vi "StiffnessTest.vi"(8 "error in (no error)":errorcluster, 10 "Model in":refnum<class "Model.lvclass">, 11 "Test Actuator State in":refnum<class "Test Actuator State.lvclass">) -> (0 "error out":errorcluster, 2 "Model out":refnum<class "Model.lvclass">, 3 "Test Actuator State out":refnum<class "Test Actuator State.lvclass">)   [LabVIEW 2016, in "Test Actuator State.lvclass"]
uses:
  Test Actuator State.lvclass
  Model/Model/Model.lvclass
  Typedefs/TestStatus.ctl
  Model/Model/Model.lvclass/Model.ctl
  Typedefs/HPMT_Typedefs.lvlib
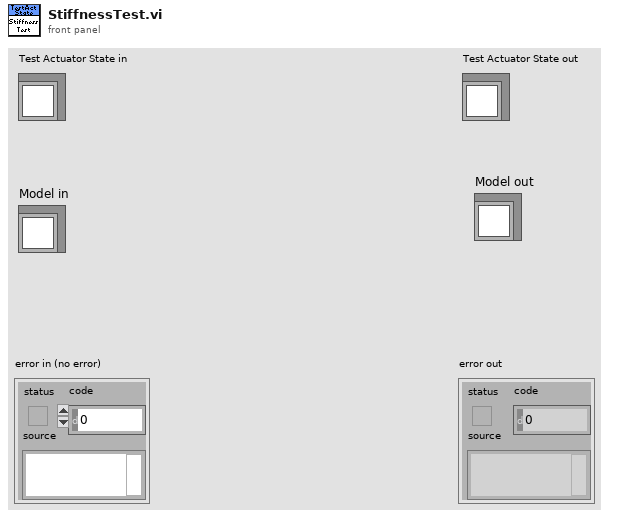
[diagram p1: front panel]
types:
  T1 = typedef "HPMT_Typedefs.lvlib/TestStatus.ctl" = enum16{"Not Run", "Running", "Passed", "Failed"}
  T2 = typedef "HPMT_Typedefs.lvlib/AllTestStatus.ctl" = cluster{"Stiffness Test":T1}
  T3 = typedef "HPMT_Typedefs.lvlib/TestSettings.ctl" = cluster{"Operator":string, "Strut Number":string, "Test Stand Serial Number":string, "Notes":string, "Test Angle":u16, "Number of Cycles":u16, "Data Points per Cycle":u16, "Settling Time (secs)":u16, "Breakaway Air Pressure":u16, "Largest Strut Displacement":dbl, "Load Cell Sensitivity":dbl, "Micron to Step Ratio":dbl}
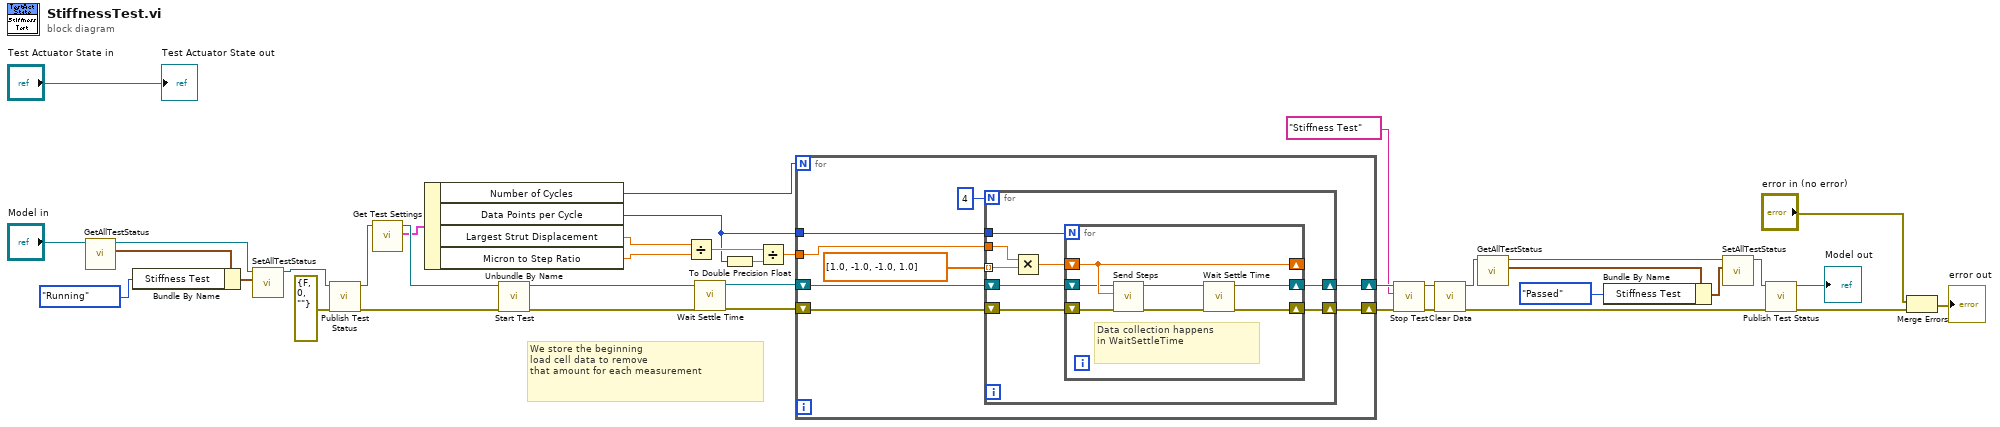
[diagram p0: block diagram]
diagram:
  # "We store the beginning\nload cell data to remove\nthat amount for each measurement"
  n1 = call "GetAllTestStatus.vi"("Model in"="Model in") -> ("AllTestStatus"=w39:T2, "Model out"=w37:refnum<class "Model.lvclass">)  [unwired: 9 in]
  n2 = Bundle By Name(cluster=w39, "Stiffness Test"=TestStatus."Running" ("TestStatus")) -> (w38:T2)
  n3 = call "SetAllTestStatus.vi"("AllTestStatus"=w38, "Model in"=w37) -> ("Model out"=w36:refnum<class "Model.lvclass">)  [unwired: 9 in]
  n4 = call "Publish Test Status.vi"("error in (no error)"=errorcluster {"status"=FALSE, "code"=0, "source"=""} ("error constant"), "Model in"=w36) -> ("error out"=w13:errorcluster, "Model out"=w15:refnum<class "Model.lvclass">)  [unwired: 8 in]
  n5 = call "Get Test Settings.vi"("Model in"=w15) -> ("Test Settings"=w12:T3, "Model out"=w14:refnum<class "Model.lvclass">)  [unwired: 9 in]
  n6 = Unbundle By Name(w12) -> ("Number of Cycles"=w11:u16, "Data Points per Cycle"=w6:u16, "Largest Strut Displacement"=w10:dbl, "Micron to Step Ratio"=w5:dbl)
  n7 = call "Start Test.vi"("error in (no error)"=w13, "Model in"=w14) -> ("error out"=w3:errorcluster, "Model out"=w4:refnum<class "Model.lvclass">)  [unwired: 8 in]
  n8 = Divide(x=w10, y=w5) -> (x/y=w9:dbl)
  n9 = call "Wait Settle Time.vi"("error in (no error)"=w3, "Model in"=w4) -> ("error out"=w1:errorcluster, "Model out"=w2:refnum<class "Model.lvclass">)  [unwired: 8 in]
  n10 = To Double Precision Float(number=w6) -> (double precision float=w7:dbl)
  n11 = Divide(x=w9, y=w7) -> (x/y=w8:dbl)
  n12 = for {
    N: w11 -> [_]
    shift-right: [w45] -> w32
    shift-left: w2 -> [w47]
    shift-right: [w44] -> w31
    shift-left: w1 -> [w46]
    tunnel: w8 -> [w41]
    tunnel: w6 -> [w40]
    n13 = for {
      N: 4 -> [_]
      shift-right: [w53] -> w45
      shift-left: w47 -> [w55]
      shift-right: [w52] -> w44
      shift-left: w46 -> [w54]
      tunnel: dbl[] [1.0, -1.0, -1.0, 1.0] -> [w51] mode=indexing
      tunnel: w41 -> [w50]
      tunnel: w40 -> [w48]
      n14 = Multiply(x=w50, y=w51) -> (x*y=w49:dbl)
      n15 = for {
        N: w48 -> [_]
        shift-right: [w61] -> w53
        shift-left: w55 -> [w59]
        shift-right: [w60] -> w52
        shift-left: w54 -> [w58]
        shift-right: [w62] -> _
        shift-left: w49 -> [w62]
        # "Data collection happens\nin WaitSettleTime"
        n16 = call "Send Steps.vi"("error in (no error)"=w58, "Command.Steps"=w62, "Model in"=w59) -> ("error out"=w56:errorcluster, "Model out"=w57:refnum<class "Model.lvclass">)  [unwired: 7 in]
        n17 = call "Wait Settle Time.vi"("error in (no error)"=w56, "Model in"=w57) -> ("error out"=w60:errorcluster, "Model out"=w61:refnum<class "Model.lvclass">)  [unwired: 8 in]
      }
    }
  }
  n18 = call "Stop Test.vi"("error in (no error)"=w31, "Test"="Stiffness Test", "Model in"=w32) -> ("error out"=w34:errorcluster, "Model out"=w33:refnum<class "Model.lvclass">)  [unwired: 7 in]
  n19 = call "Clear Data.vi"("error in (no error)"=w34, "Model in"=w33) -> ("error out"=w29:errorcluster, "Model out"=w27:refnum<class "Model.lvclass">)  [unwired: 8 in]
  n20 = call "GetAllTestStatus.vi"("Model in"=w27) -> ("AllTestStatus"=w26:T2, "Model out"=w24:refnum<class "Model.lvclass">)  [unwired: 9 in]
  n21 = Bundle By Name(cluster=w26, "Stiffness Test"=TestStatus."Passed" ("TestStatus")) -> (w25:T2)
  n22 = call "SetAllTestStatus.vi"("AllTestStatus"=w25, "Model in"=w24) -> ("Model out"=w28:refnum<class "Model.lvclass">)  [unwired: 9 in]
  n23 = call "Publish Test Status.vi"("error in (no error)"=w29, "Model in"=w28) -> ("error out"=w30:errorcluster, "Model out"=→"Model out":refnum<class "Model.lvclass">)  [unwired: 8 in]
  n24 = Merge Errors("error in (no error)", w30) -> (→"error out":errorcluster)
  "Test Actuator State out" <- "Test Actuator State in"
